vi "tlc_Initialize.vi"(6 "Play Structure Names":T1, 7 "Number of Channels":cluster{"Rows":i32, "Columns":i32}, 8 "error in (no error)":errorcluster, 9 "tlc_Consumer Queue Reference.ctl":T2, 10 "tlc_Display Queue Reference.ctl":T3, 11 "tlc_User Event Reference.ctl":T4) -> (0 "error out":errorcluster)   [LabVIEW 2018]
uses:
  Controls/tlc_User Event Reference.ctl
  Controls/tlc_Display Queue Reference.ctl
  Controls/tlc_User Interface Command.ctl
  Controls/tlc_User Interface Data Type.ctl
  Controls/tlc_Consumer Queue Reference.ctl
  Controls/tlc_Consumer Control.ctl
  Controls/tlc_Functions.ctl
  Controls/Play Structure Names.ctl
  Modules/Display/tlc_Display_Command Control.ctl
  Modules/Error/tlc_Error Module Command Control.ctl
  Modules/Cue/tlc_Cue_Information Command.ctl
  Modules/File/tlc_File_Command Control.ctl
  Modules/Hardware/tlc_Hardware_Command Control.ctl
  Modules/Timing/tlc_Timing Command Control.ctl
  Modules/Timing/tlc_Timing Stop Module Control.ctl
panel:
  # "Input"
  # "Output"
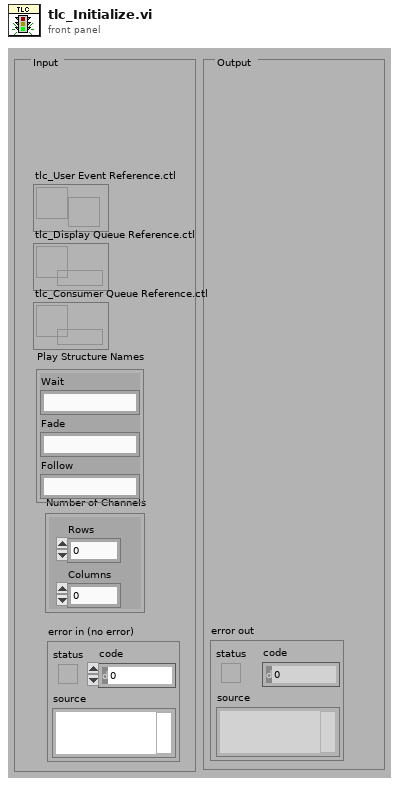
[diagram p1: front panel]
types:
  T1 = typedef "Play Structure Names.ctl" = cluster{"Wait":string, "Fade":string, "Follow":string}
  T2 = typedef "tlc_Consumer Queue Reference.ctl" = refnum<queue>
  T3 = typedef "tlc_Display Queue Reference.ctl" = refnum<queue>
  T4 = typedef "tlc_User Event Reference.ctl" = refnum<user-event>
  T5 = typedef "tlc_User Interface Data Type.ctl" = enum16{"Initialize", "Initialize Front Panel", "Update Front Panel Channels", "Select Cue in Cue List", "Enable/Disable Front Panel Controls", "Update Cue List", "Stop"}
  T6 = typedef "tlc_Timing Stop Module Control.ctl" = enum16{"Intialize", "Stop"}
  T7 = typedef "tlc_Timing Command Control.ctl" = enum16{"Initialize", "Get Information", "Create", "Wait", "Fade", "Follow", "Shutdown"}
  T8 = typedef "tlc_Hardware_Command Control.ctl" = enum16{"Initialize", "Write", "Shutdown"}
  T9 = typedef "tlc_File_Command Control.ctl" = enum16{"Initialize", "Save Cues", "Load Cues", "Shutdown"}
  T10 = typedef "tlc_Cue_Information Command.ctl" = enum16{"Add Cue", "Delete Cue", "Get Cue Values", "Set Cue Values", "Swap", "Get Number of Cues", "Initialize", "Get Empty Cue"}
  T11 = typedef "tlc_Error Module Command Control.ctl" = enum16{"Initialize", "Handle Errors", "Report Errors"}
  T12 = typedef "tlc_Display_Command Control.ctl" = enum16{"Initialize", "Update UI", "Shutdown"}
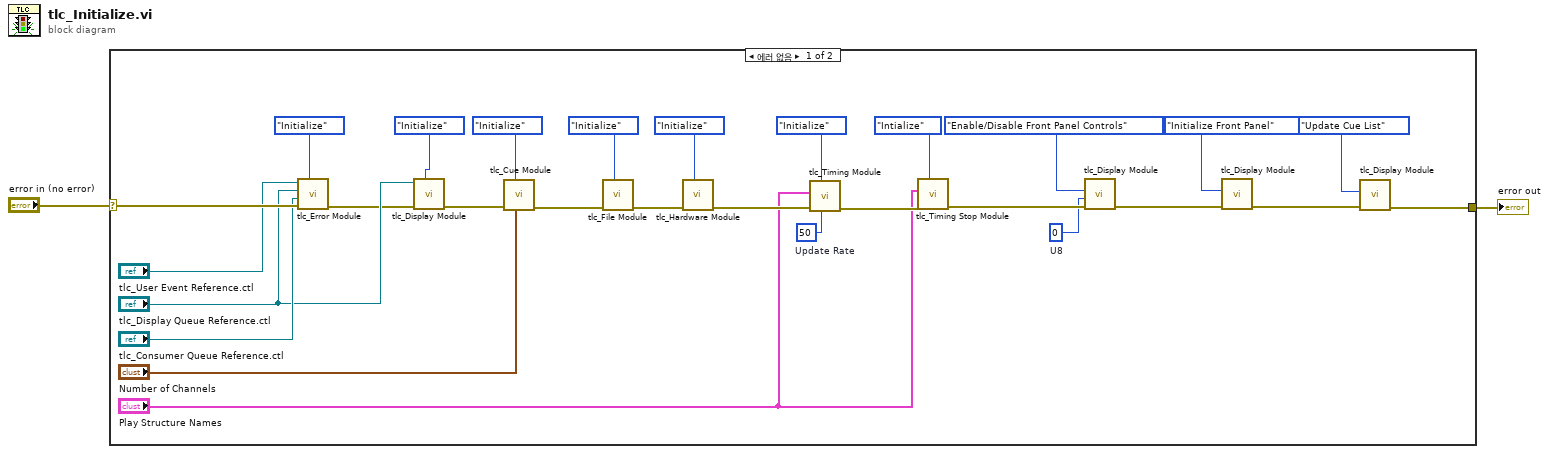
[diagram p0: block diagram]
diagram:
  n1 = case shown="에러 없음" "error in (no error)" {
    selector: "error in (no error)" -> [w30 w31]
    tunnel: [w8 w31] -> w1
    frame No Error {
      w4 = u8 0  # U8
      w5 = u32 50  # Update Rate
      n2 = call "tlc_Error Module.vi"("Command (Handle Errors"=tlc_Error_Module_Command_Control."Initialize", "error in (no error)"=w30, "tlc_Consumer Queue Reference.ctl"="tlc_Consumer Queue Reference.ctl", "tlc_Display Queue Reference.ctl"="tlc_Display Queue Reference.ctl", "tlc_User Event Reference.ctl"="tlc_User Event Reference.ctl") -> ("error out"=w25:errorcluster)  [unwired: 5 in, 1 out]
      n3 = call "tlc_Display Module.vi"("Command (Update UI)"=tlc_Display_Command_Control."Initialize", "error in (no error)"=w25, "tlc_Display Queue Reference.ctl"="tlc_Display Queue Reference.ctl") -> ("error out"=w23:errorcluster)  [unwired: 8 in]
      n4 = call "tlc_Cue Module.vi"("Number of Channels"="Number of Channels", "Command"=tlc_Cue_Information_Command."Initialize", "error in (no error)"=w23) -> ("error out"=w21:errorcluster)  [unwired: 5 in, 2 out]
      n5 = call "tlc_File Module.vi"("Command"=tlc_File_Command_Control."Initialize", "error in (no error)"=w21) -> ("error out"=w19:errorcluster)  [unwired: 8 in, 1 out]
      n6 = call "tlc_Hardware Module.vi"("Command (Write)"=tlc_Hardware_Command_Control."Initialize", "error in (no error)"=w19) -> ("error out"=w17:errorcluster)  [unwired: 9 in]
      n7 = call "tlc_Timing Module.vi"("Update Rate"=w5, "Command"=tlc_Timing_Command_Control."Initialize", "error in (no error)"=w17, "Play Structure Names"="Play Structure Names") -> ("error out"=w15:errorcluster)  [unwired: 5 in, 2 out]
      n8 = call "tlc_Timing Stop Module.vi"("Command (Stop)"=tlc_Timing_Stop_Module_Control."Intialize", "error in (no error)"=w15, "Play Structure Names"="Play Structure Names") -> ("error out"=w13:errorcluster)  [unwired: 8 in]
      n9 = call "tlc_Display Module.vi"("error in (no error)"=w13, "Data"=w4, "Data Type"=tlc_User_Interface_Data_Type."Enable/Disable Front Panel Controls") -> ("error out"=w11:errorcluster)  [unwired: 8 in]
      n10 = call "tlc_Display Module.vi"("error in (no error)"=w11, "Data Type"=tlc_User_Interface_Data_Type."Initialize Front Panel") -> ("error out"=w9:errorcluster)  [unwired: 9 in]
      n11 = call "tlc_Display Module.vi"("error in (no error)"=w9, "Data Type"=tlc_User_Interface_Data_Type."Update Cue List") -> ("error out"=w8:errorcluster)  [unwired: 9 in]
    }
    frame Error {
    }
  }
  "error out" <- w1
